vi "1WIRE_wait for convert.vi"(7 "1-Wire DIO Pin":refnum<k21>="ConnectorA/DIO15", 8 "error in":errorcluster) -> (0 "error out":errorcluster, 3 "Convert Time (usec)":u32)   [LabVIEW 2014]
doc: "This VI is created by Vincent Claes for FPDA-1 more information on http://pwo.fpga.be\n\nvincent.claes@xios.be\nclaesvincent@gmail.com\n\nhttp://www.linkedin.com/in/vincentclaes"
uses:
  <vilib>/rvi/Emulation/niFpgaGetClockAttributes.vi
  <vilib>/rvi/Emulation/niFpgaSctlEmulationGetInTimedLoop.vi
  <vilib>/rvi/Emulation/niFpgaEmulationReportErrorSimple.vi
  <vilib>/rvi/Emulation/niFpgaCriticalErrorInLSC.vi
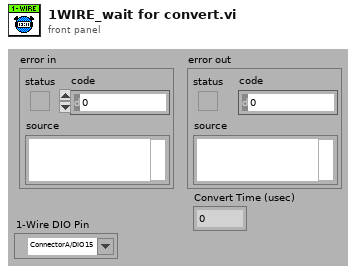
[diagram p1: front panel]
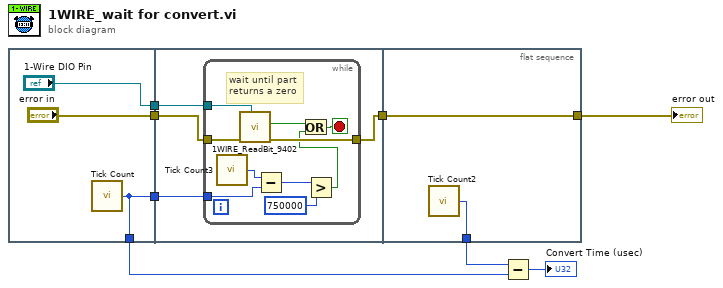
[diagram p0: block diagram]
diagram:
  n1 = flat-sequence {
    tunnel: ["error in"] -> w7
    tunnel: [w10] -> w4
    tunnel: [w10] -> w2
    tunnel: ["1-Wire DIO Pin"] -> w1
    tunnel: w7 -> [w15]
    tunnel: [w14] -> w6
    tunnel: w2 -> [w13]
    tunnel: w1 -> [w12]
    tunnel: [w27] -> w8
    tunnel: w6 -> [w27]
    tunnel: [w26] -> w5
    frame #0 {
      n2 = call "Tick Count"() -> ("Tick Count(uSec)"=w10:u32)
    }
    frame #1 {
      n3 = while {
        tunnel: w15 -> [w25]
        tunnel: [w23] -> w14
        tunnel: w13 -> [w21]
        tunnel: w12 -> [w16]
        stop <- w20 stop-if-true
        # "wait until part\nreturns a zero"
        n4 = call "Tick Count3"() -> ("Tick Count(uSec)"=w22:u32)
        n5 = call "1WIRE_ReadBit_9402.vi"("1-Wire DIO Pin"=w16, "error in"=w25) -> ("error out"=w23:errorcluster, "Bit Read"=w24:bool)  [unwired: 8 in]
        n6 = Subtract(x=w22, y=w21) -> (x-y=w18:u32)
        n7 = Greater?(x=w18, y=u32 750000 ("x")) -> (0:w19:bool)
        n8 = Or(x=w24, y=w19) -> (x .or. y?=w20:bool)
      }
    }
    frame #2 {
      n9 = call "Tick Count2"() -> ("Tick Count(uSec)"=w26:u32)
    }
  }
  n10 = Subtract(x=w5, y=w4) -> (x-y=→"Convert Time (usec)":u32)
  "error out" <- w8
